vi "ErrorObstruccion.vi"(1 "Buffer Overflow":bool) -> (0 "error out":errorcluster)   [LabVIEW 2015]
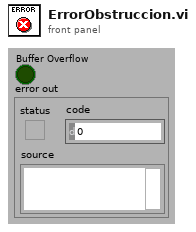
[diagram p1: front panel]
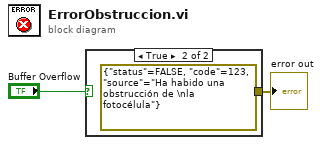
[diagram p0: block diagram]
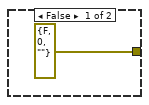
[diagram p2: hidden frame]
diagram:
  n1 = case shown="True" "Buffer Overflow" {
    tunnel: [errorcluster {"status"=FALSE, "code"=0, "source"=""} ("error out") errorcluster {"status"=FALSE, "code"=123, "source"="Ha habido una obstrucción de \nla fotocélula"} ("error out")] -> w1
    frame False {
    }
    frame True {
    }
  }
  "error out" <- w1
